vi "Teardown.vi"(8 "Error In":errorcluster, 10 "Known Host":refnum<class "Known Host.lvclass">, 11 "Known Hosts":refnum<class "Known Hosts.lvclass">) -> (0 "Error Out":errorcluster)   [LabVIEW 2018, in "Tests.lvlib" / "Known Host.lvlib"]
uses:
  Known Host.lvlib
  src/Toolkit/Known Host/Known Host.lvclass
  src/Toolkit/Known Hosts/Known Hosts.lvclass
  src/Toolkit/Known Host/Support/Destroy to Known Hosts.vi
  src/Toolkit/Known Hosts/Support/Destroy to Session.vi
  src/Toolkit/Session/Support/Destroy to SSH.vi
  src/Toolkit/Session/Session.lvclass
  src/Toolkit/SSH/SSH.lvclass
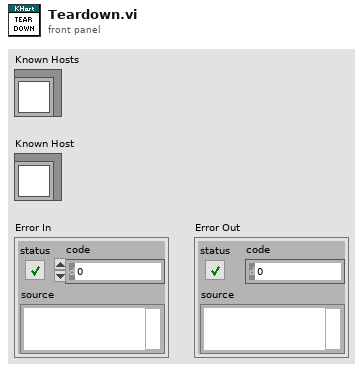
[diagram p1: front panel]
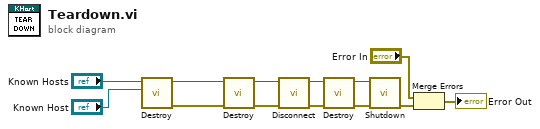
[diagram p0: block diagram]
diagram:
  n1 = call-poly "Destroy.vi"("Known Host"="Known Host", "KnownHosts In"="Known Hosts") -> ("Error Out"=w4:errorcluster, "KnownHosts Out"=w2:refnum<class "Known Hosts.lvclass">)  [unwired: 8 in]
  n2 = call-poly "Destroy.vi"("Error In"=w4, "Known Hosts"=w2) -> ("Error Out"=w8:errorcluster, "Session"=w5:refnum<class "Session.lvclass">)  [unwired: 8 in]
  n3 = call "Disconnect.vi"("Error In"=w8, "Session In"=w5) -> ("Error Out"=w13:errorcluster, "Sesssion Out"=w12:refnum<class "Session.lvclass">)  [unwired: 8 in]
  n4 = call-poly "Destroy.vi"("Error In"=w13, "Session"=w12) -> ("Error Out"=w10:errorcluster, "SSH"=w9:refnum<class "SSH.lvclass">)  [unwired: 8 in]
  n5 = call "Shutdown.vi"("Error In"=w10, "SSH"=w9) -> ("Error Out"=w11:errorcluster)  [unwired: 9 in]
  n6 = Merge Errors("Error In", w11) -> (→"Error Out":errorcluster)
